vi "Get a Voltage by ENUM.vi"(9 "DMM Voltages":dbl[](array[numeric]), 11 "Selector":T1(ring)) -> (3 "Measurement":dbl)   [LabVIEW 2015]
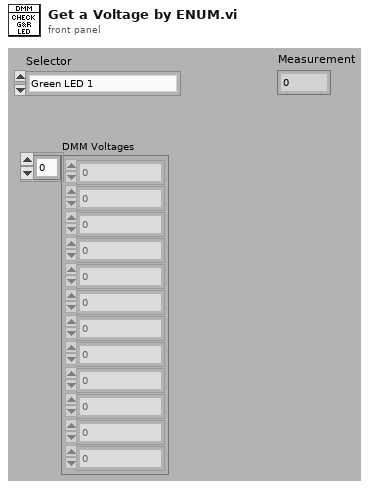
[diagram p1: front panel]
types:
  T1 = enum16{"Green LED 1", "Red LED", "VCELL", "VP2 TESTER", "TEMP TESTER", "Green LED 2"}
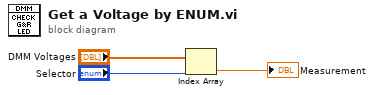
[diagram p0: block diagram]
diagram:
  n1 = Index Array(array="DMM Voltages", index="Selector") -> (element=→"Measurement":dbl)
